vi "HandleNotifications.vi"(8 "error in (no error)":errorcluster, 11 "navX - Interface in":refnum<class "navX - Interface.lvclass">) -> (0 "error out":errorcluster, 1 "Halt?":bool, 3 "navX - Interface out":refnum<class "navX - Interface.lvclass">)   [LabVIEW 2015, in "navX Library v3.lvlib" / "navX - Interface.lvclass"]
uses:
  navX - Interface.lvclass
  navX - Interface.lvclass/navX - Interface.ctl
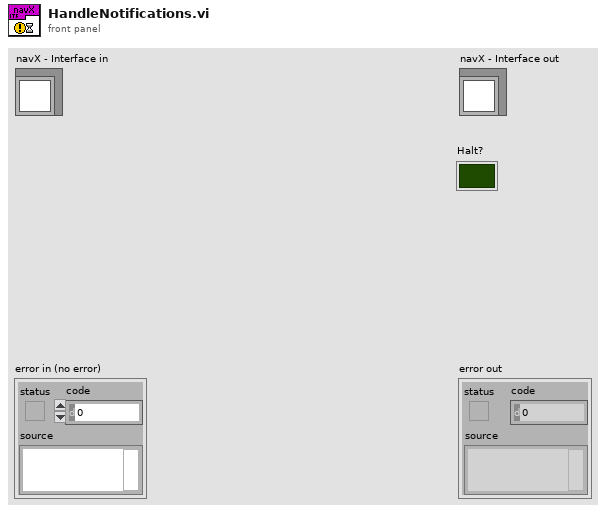
[diagram p1: front panel]
types:
  T1 = typedef "navX Library v3.lvlib/navX - Interface.lvclass/NotificationPacketTypeDef.ctl" = cluster{"Notification Action":T2, "Notification Data":variant}
  T2 = typedef "navX Library v3.lvlib/navX - Interface.lvclass/NotificationActionsTypeDef.ctl" = enum16{"UNKNOWN", "Stop Processing Loop", "Reconfigure", "Zero"}
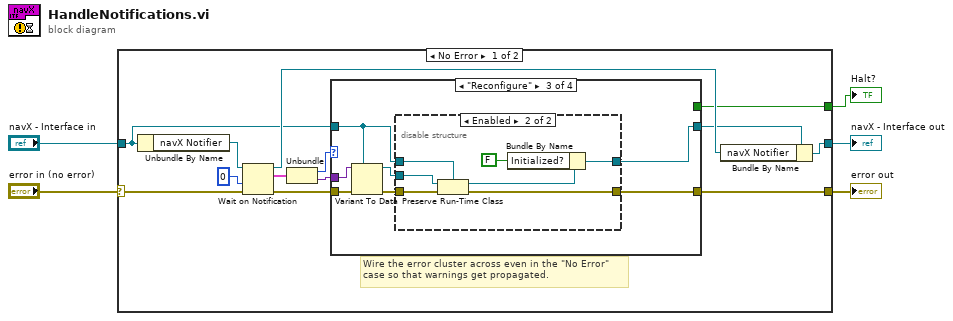
[diagram p0: block diagram]
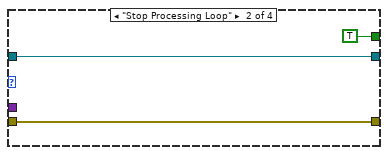
[diagram p3: hidden frame]
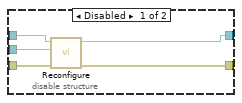
[diagram p4: hidden frame]
diagram:
  n1 = case shown="No Error" "error in (no error)" {
    selector: "error in (no error)" -> [w14 w46]
    tunnel: [w6 w46] -> w4
    tunnel: [w18 w45] -> w2
    tunnel: "navX - Interface in" -> [w11 w45]
    tunnel: [w9 _] -> w1
    frame No Error {
      # "Wire the error cluster across even in the \"No Error\"\ncase so that warnings get propagated."
      n2 = Unbundle By Name(w11) -> ("navX Notifier"=w17:refnum<notifier>)
      n3 = Wait on Notification(notifier=w17, timeout in ms (-1)=0, error in (no error)=w14) -> (notifier out=w16:refnum<notifier>, notification=w13:T1, error out=w7:errorcluster)  [unwired: 1 in, 1 out]
      n4 = Unbundle(w13) -> ("Notification Action"=w12:T2, "Notification Data"=w8:variant)
      n5 = case shown="\"Reconfigure\"" w12 {
        tunnel: [w20 w23 w24 w44] -> w10
        tunnel: w11 -> [w20 w23 w26 w44]
        tunnel: [_ TRUE _ _] -> w9
        tunnel: w8 -> [_ _ w30 _]
        tunnel: w7 -> [w19 w21 w29 w43]
        tunnel: [w19 w21 w27 w43] -> w6
        frame "UNKNOWN", Default {
        }
        frame "Stop Processing Loop" {
        }
        frame "Reconfigure" {
          n6 = Variant To Data(error in=w29, type=w26, Variant=w30) -> (data=w25:refnum<class "navX - Interface.lvclass">, error out=w28:errorcluster)
          n7 = disable-structure shown="Enabled" {
            disable-tunnel: w28 -> [w35 w41]
            disable-tunnel: [w34 w39] -> w27
            disable-tunnel: w26 -> [w33 w40]
            disable-tunnel: w25 -> [w32 w42]
            disable-tunnel: [w31 w37] -> w24
            frame Disabled {
              n8 = call-dynamic "Reconfigure.vi"("error in (no error)"=w35, "navX - Interface Update in"=w32, "navX - Interface in"=w33) -> ("error out"=w34:errorcluster, "navX - Interface out"=w31:refnum<class "navX - Interface.lvclass">)  [unwired: 7 in]
            }
            frame Enabled {
              n9 = Preserve Run-Time Class(object in=w42, error in=w41, 2:w40) -> (object out=w38:refnum<class "navX - Interface.lvclass">, error out=w39:errorcluster)
              n10 = Bundle By Name(cluster=w38, "Initialized?"=FALSE) -> (w37:refnum<class "navX - Interface.lvclass">)
            }
          }
        }
        frame "Zero" {
        }
      }
      n11 = Bundle By Name(cluster=w10, "navX Notifier"=w16) -> (w18:refnum<class "navX - Interface.lvclass">)
    }
    frame Error {
    }
  }
  "error out" <- w4
  "navX - Interface out" <- w2
  "Halt?" <- w1
